vi "点阵图标定-烧.vi"() -> ()   [LabVIEW 2018]
uses:
  <vilib>/vision/Calibration.llb/Distortion Model.ctl
  <vilib>/vision/Calibration.llb/Distortion Model Types.ctl
  <vilib>/vision/NI_Vision_Development_Module.lvlib
panel:
  out "ROI Descriptor":T1 {"Contours"."Type" items=["No Selection", "Point", "Line", "Rectangle", "Oval", "Polygon", "Freehand Region", "Annulus", "Unused2", "Unused3", "Broken Line", "Freehand Line", "Rotated Rectangle"]}
  in  "刷新按钮":bool
  in  "停止按钮":bool
  in  "确定按钮":bool
  in  "标定系数设置":cluster{"X轴方向间距":sgl, "Y轴方向间距":sgl, "单位选择":u16} {"单位选择" items=["Undefined", "Angstrom", "Micrometer", "Millimeter", "Centimeter", "Meter", "Kilometer", "Microinch", "Inch", "Feet", "Nautical miles", "Standardmiles", "Steps"]}
  out "二值化点阵图":T2(plugin-control)
  out "点阵图":T2(plugin-control)
  # "点阵图标定"
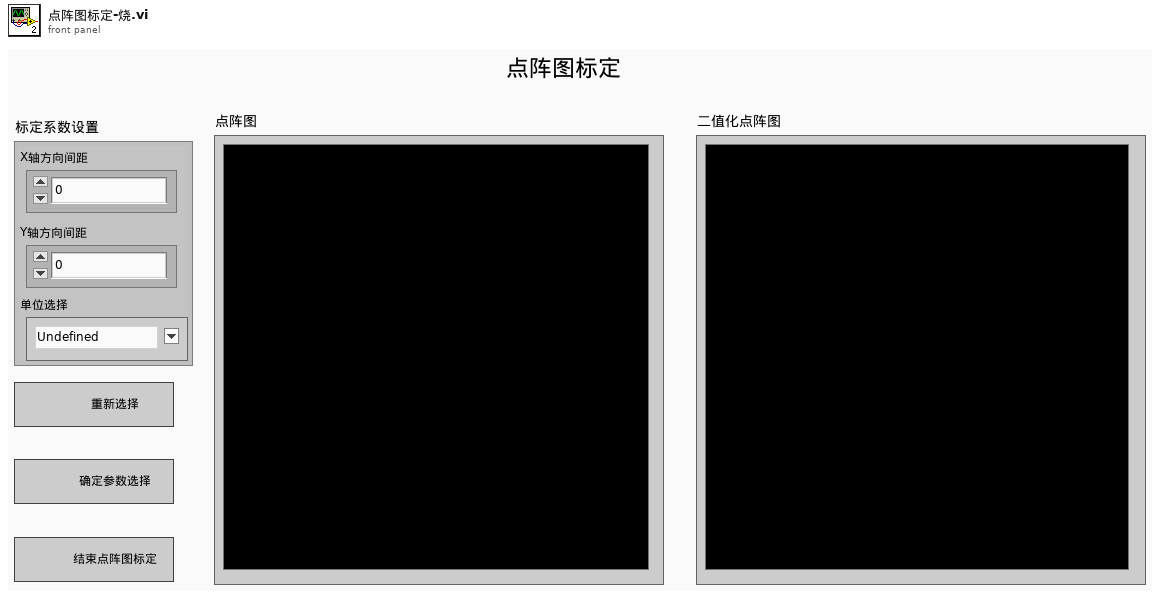
[diagram p1: front panel]
types:
  T1 = typedef "ROI Descriptor" = cluster{"Global Rectangle":i32[], "Contours":cluster{"ID":enum32{"External", "Internal"}, "Type":u32, "Coordinates":i32[]}[]}
  T2 = typedef "IMAQ Image.ctl" = refnum<image>
  T3 = enum8{"Enabled", "Disabled", "Disabled and Grayed Out"}
  T4 = enum32{"Invalid", "Standard", "Closed", "Hidden", "Minimized", "Maximized"}
  T5 = typedef "Image Type" = u32
  T6 = typedef "IMAQ Rectangle" = cluster{"Left":i32, "Top":i32, "Right":i32, "Bottom":i32, "Rotation":dbl}
  T7 = typedef "Distortion Model.ctl" = cluster{"Distortion Model":T8, "Polynomial Model Setup":cluster{"Radial Coefficient":u32, "Tangential Coefficients ":bool}}
  T8 = typedef "Distortion Model Types.ctl" = i32
  T9 = typedef "Calibration Reference Points.ctl" = cluster{"Pixel Coordinates":cluster{"X":dbl, "Y":dbl}[], "Real World Coordinates":cluster{"X":dbl, "Y":dbl}[], "Unit":T10, "Image Size":cluster{"X":u32, "Y":u32}}
  T10 = typedef "Image Unit" = enum32{"Undefined", "Angström", "Micrometer", "Millimeter", "Centimeter", "Meter", "Kilometer", "Microinch", "Inch", "Feet", "Nautical miles", "Standard miles", "Steps"}
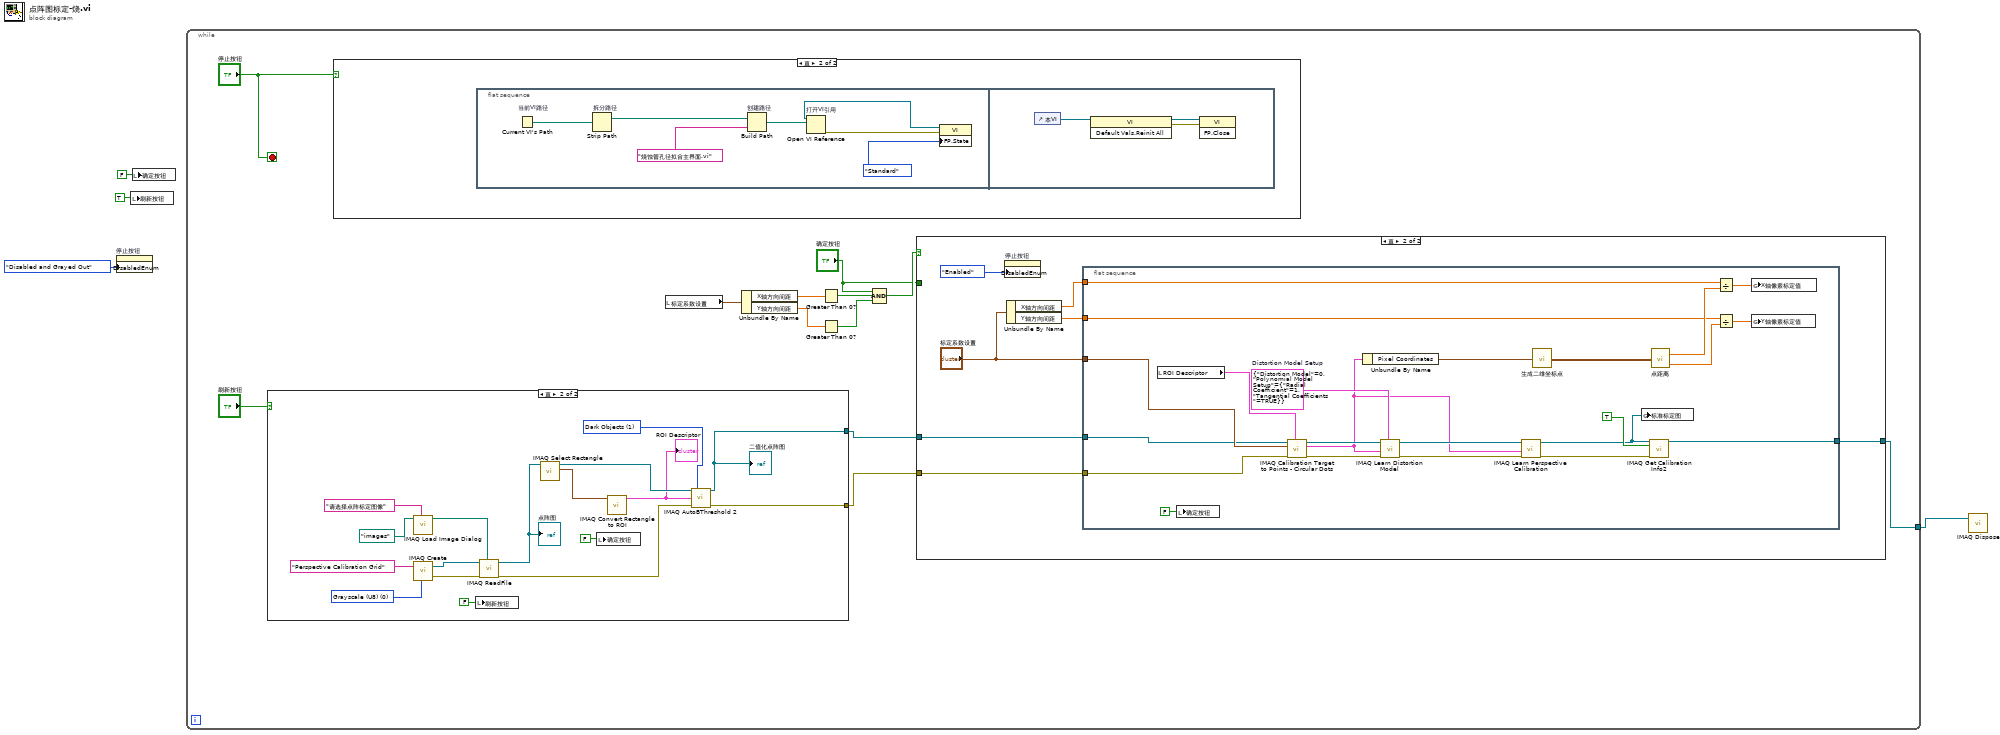
[diagram p0: block diagram]
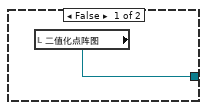
[diagram p2: hidden frame]
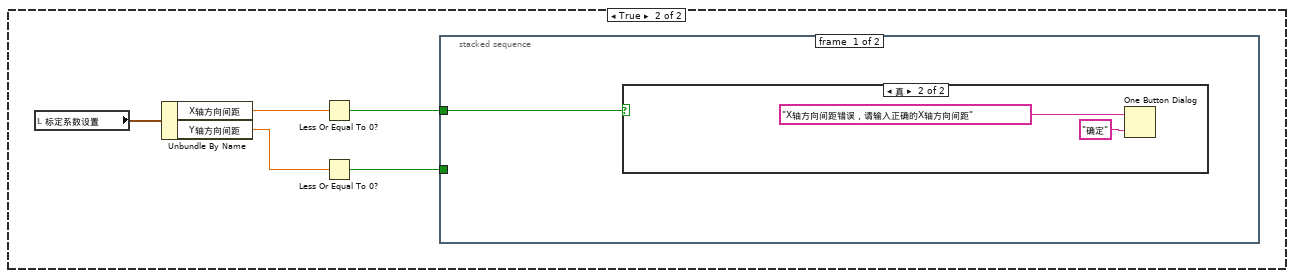
[diagram p5: hidden frame]
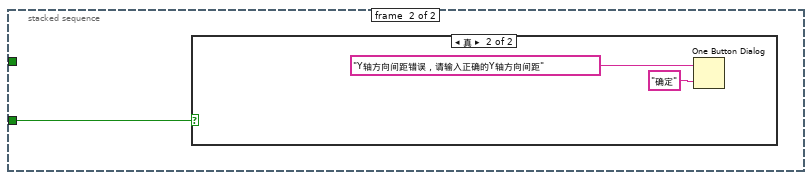
[diagram p7: hidden frame]
diagram:
  n1 = property on="停止按钮" class="Bool"("DisabledEnum"=T3."Disabled and Grayed Out" ("禁用")) -> ()  [unwired: 2 in, 2 out]
  n2 = local write "刷新按钮"(TRUE ("刷新按钮")) -> ()
  n3 = local write "确定按钮"(FALSE ("确定按钮")) -> ()
  n4 = while {
    tunnel: [w16] -> w2
    stop <- "停止按钮" stop-if-true
    n5 = case shown="真" "刷新按钮" {
      tunnel: [w17 w23] -> w14
      tunnel: [_ w25] -> w13
      frame False {
        n6 = local read "二值化点阵图"() -> (w17:T2)
      }
      frame True {
        w34 = u32 1 items=["Bright Objects", "Dark Objects"] ("Look For (Bright Objects)")
        w32 = T5 0 items=["Grayscale (U8)", "Grayscale (I16)", "Grayscale (SGL)", "Complex (CSG)", "RGB (U32)", "HSL (U32)", "RGB (U64)", "Grayscale (U16)"] ("Image Type")
        n7 = call "IMAQ Load Image Dialog"("Prompt"="请选择点阵标定图像" ("prompt"), "Start Path"=path "images") -> ("Path"=w30:path)  [unwired: 7 in, 2 out]
        n8 = call "IMAQ Create"("Image Name"="Perspective Calibration Grid", "Image Type"=w32) -> ("New Image"=w27:T2, "error out"=w28:errorcluster)  [unwired: 2 in, 1 out]
        n9 = local write "刷新按钮"(FALSE ("刷新按钮")) -> ()
        n10 = call "IMAQ ReadFile"("File Path"=w30, "error in (no error)"=w28, "Image"=w27) -> ("error out"=w33:errorcluster, "Image Out"=w21:T2)  [unwired: 2 in, 5 out]
        "点阵图" <- w21
        n11 = call "IMAQ Select Rectangle"("Image In"=w21) -> ("Rectangle"=w19:T6, "Image Out (duplicate)"=w20:T2)  [unwired: 7 in, 2 out]
        n12 = local write "确定按钮"(FALSE ("刷新按钮")) -> ()
        n13 = call "IMAQ Convert Rectangle to ROI"("Rectangle"=w19) -> ("ROI Descriptor"=w18:T1)  [unwired: 8 in, 1 out]
        "ROI Descriptor" <- w18
        n14 = call "IMAQ AutoBThreshold 2"("Image Src"=w20, "Look For (Bright Objects)"=w34, "ROI Descriptor"=w18, "error in (no error)"=w33) -> ("Image Dst Out"=w23:T2, "error out"=w25:errorcluster)  [unwired: 9 in, 1 out]
        "二值化点阵图" <- w23
      }
    }
    n15 = case shown="真" "停止按钮" {
      frame False {
      }
      frame True {
        n16 = flat-sequence {
          frame #0 {
            n17 = Current VI's Path "当前VI路径"() -> (path=w39:path)
            n18 = Strip Path "拆分路径"(path=w39) -> (stripped path=w41:path)  [unwired: 1 out]
            n19 = Build Path "创建路径"(base path=w41, name or relative path="烧蚀管孔径拟合主界面.vi" ("名称或相对路径")) -> (appended path=w40:path)
            n20 = Open VI Reference "打开VI引用"(vi path=w40) -> (vi reference=w38:refnum<vi>, error out=w37:errorcluster)  [unwired: 5 in]
            n21 = property class="VI"(reference=w38, error in=w37, "FP.State"=T4."Standard" ("前面板窗口:状态")) -> ()  [unwired: 2 out]
          }
          frame #1 {
            n22 = control-ref of="本VI"() -> (w42:refnum<vi>)
            n23 = invoke class="VI" method="Default Vals.Reinit All"(reference=w42) -> (reference out=w43:refnum<vi>, error out=w44:errorcluster)  [unwired: 2 in, 1 out]
            n24 = invoke class="VI" method="FP.Close"(reference=w43, error in=w44) -> ()  [unwired: 1 in, 3 out]
          }
        }
      }
    }
    n25 = local read "标定系数设置"() -> (w11:cluster{"X轴方向间距":sgl, "Y轴方向间距":sgl, "单位选择":u16})
    n26 = Unbundle By Name(w11) -> ("X轴方向间距"=w10:sgl, "Y轴方向间距"=w9:sgl)
    n27 = Greater Than 0?(x=w10) -> (x > 0?=w7:bool)
    n28 = Greater Than 0?(x=w9) -> (x > 0?=w6:bool)
    n29 = Compound Arithmetic op=AND("确定按钮", w7, w6) -> (w8:bool)
    n30 = case shown="真" w8 {
      tunnel: [_ w57] -> w16
      tunnel: w14 -> [_ w63]
      tunnel: w13 -> [_ w62]
      tunnel: "确定按钮" -> [w45 _]
      frame False {
        n31 = case shown="假" w45 {
          frame False {
          }
          frame True {
            n32 = local read "标定系数设置"() -> (w50:cluster{"X轴方向间距":sgl, "Y轴方向间距":sgl, "单位选择":u16})
            n33 = Unbundle By Name(w50) -> ("X轴方向间距"=w49:sgl, "Y轴方向间距"=w47:sgl)
            n34 = Less Or Equal To 0?(x=w49) -> (x <= 0?=w48:bool)
            n35 = Less Or Equal To 0?(x=w47) -> (x <= 0?=w46:bool)
            n36 = stacked-sequence {
              tunnel: w48 -> [w51 _]
              tunnel: w46 -> [_ w54]
              frame #0 {
                n37 = case shown="真" w51 {
                  frame False {
                  }
                  frame True {
                    n38 = One Button Dialog(message="X轴方向间距错误，请输入正确的X轴方向间距" ("消息"), button name ("OK")="确定" ("按钮名称（“确定”）")) -> ()  [unwired: 1 out]
                  }
                }
              }
              frame #1 {
                n39 = case shown="真" w54 {
                  frame False {
                  }
                  frame True {
                    n40 = One Button Dialog(message="Y轴方向间距错误，请输入正确的Y轴方向间距" ("消息"), button name ("OK")="确定" ("按钮名称（“确定”）")) -> ()  [unwired: 1 out]
                  }
                }
              }
            }
          }
        }
      }
      frame True {
        n41 = property on="停止按钮" class="Bool"("DisabledEnum"=T3."Enabled" ("禁用")) -> ()  [unwired: 2 in, 2 out]
        n42 = Unbundle By Name("标定系数设置") -> ("X轴方向间距"=w59:sgl, "Y轴方向间距"=w58:sgl)
        n43 = flat-sequence {
          tunnel: "标定系数设置" -> [w79]
          tunnel: w63 -> [w77]
          tunnel: w62 -> [w76]
          tunnel: w59 -> [w70]
          tunnel: w58 -> [w69]
          tunnel: [w64] -> w57
          frame #0 {
            w83 = T7 {"Distortion Model"=0, "Polynomial Model Setup"={"Radial Coefficient"=1, "Tangential Coefficients "=TRUE}}  # Distortion Model Setup
            n44 = local read "ROI Descriptor"() -> (w75:T1)
            n45 = local write "确定按钮"(FALSE ("确定按钮")) -> ()
            n46 = call "IMAQ Calibration Target to Points - Circular Dots"("ROI Descriptor"=w75, "error in (no error)"=w76, "Grid Descriptor"=w79, "Target Image"=w77) -> ("error out"=w82:errorcluster, "Reference Points"=w74:T9, "Target Image (dup)"=w86:T2)  [unwired: 1 in, 4 out]
            n47 = Unbundle By Name(w74) -> ("Pixel Coordinates"=w73:cluster{"X":dbl, "Y":dbl}[])
            n48 = call "IMAQ Learn Distortion Model"("Distortion Model Setup"=w83, "error in (no error)"=w82, "Reference Points"=w74, "Calibration Template Image"=w86) -> ("error out"=w81:errorcluster, "Calibration Template Image Out"=w85:T2)  [unwired: 2 in, 4 out]
            n49 = call "IMAQ Learn Perspective Calibration"("error in (no error)"=w81, "Reference Points"=w74, "Calibration Template Image"=w85) -> ("error out"=w80:errorcluster, "Calibration Template Image Out"=w65:T2)  [unwired: 1 in, 6 out]
            n50 = call "生成二维坐标点.vi"("输入无序一维坐标点"=w73) -> ("输出有序二维坐标点"=w72:cluster{"X":sgl, "Y":sgl}[][])
            n51 = global write "全局变量.vi" "标准标定图"(w65) -> ()
            n52 = call "IMAQ Get Calibration Info2"("Calibration Template Image"=w65, "Return Error Information (False)"=TRUE, "error in (no error)"=w80) -> ("Calibration Template Image (duplicate)"=w64:T2)  [unwired: 12 out]
            n53 = call "点距离.vi"("二维点阵"=w72) -> ("X间距"=w71:sgl, "Y间距"=w68:sgl)
            n54 = Divide(x=w70, y=w71) -> (x/y=w67:sgl)
            n55 = Divide(x=w69, y=w68) -> (x/y=w66:sgl)
            n56 = global write "全局变量.vi" "X轴像素标定值"(w67) -> ()
            n57 = global write "全局变量.vi" "Y轴像素标定值"(w66) -> ()
          }
        }
      }
    }
  }
  n58 = call "IMAQ Dispose"("Image"=w2) -> ()  [unwired: 5 in, 1 out]
